vi "全局变量.vi"() -> ()   [LabVIEW 2022 SP3]
panel:
  out "lastENC":dbl
  out "ENC调节比例":dbl
  out "自动起摆平衡":bool
  out "积分ENC":dbl
  out "微分ENC":dbl
  out "积分ADC":dbl
  out "微分ADC":dbl
  out "ENC滤波长度":dbl
  out "ENC滤波辅助":dbl[](array[numeric])
  out "ENC滤波":dbl
  out "目标ENC":dbl
  out "获得初始ENC":bool
  in  "状态":string
  # "pidADC"
  # "pidENC"
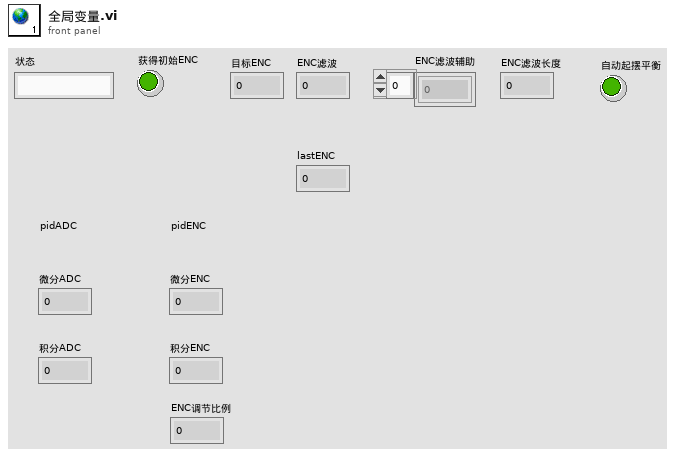
[diagram p1: front panel]
diagram:
